vi "Read FRU.vi"(0 "Device In":T2, 1 "FRU Type":T5, 2 "FRU In":T4, 5 "i2c configuration in":T3, 7 "CSV Path":path, 9 "Unique FRU Data":T1, 11 "error in (no error)":errorcluster) -> (3 "FRU Out":T4, 4 "Device Out":T2, 6 "i2c configuration out":T3, 8 "Read Byte":u8[](array[numeric]) format="%02x", 14 "PASS":bool, 15 "error out":errorcluster)   [LabVIEW 2025]
uses:
  Type Definitions/FRU Information.ctl
  <vilib>/ni845x/ni845x.llb/ni845xControl.ctl
  <vilib>/ni845x/ni845x.llb/ni845xI2cConfiguration.ctl
  Type Definitions/FRU Type.ctl
  Type Definitions/Unique FRU Input.ctl
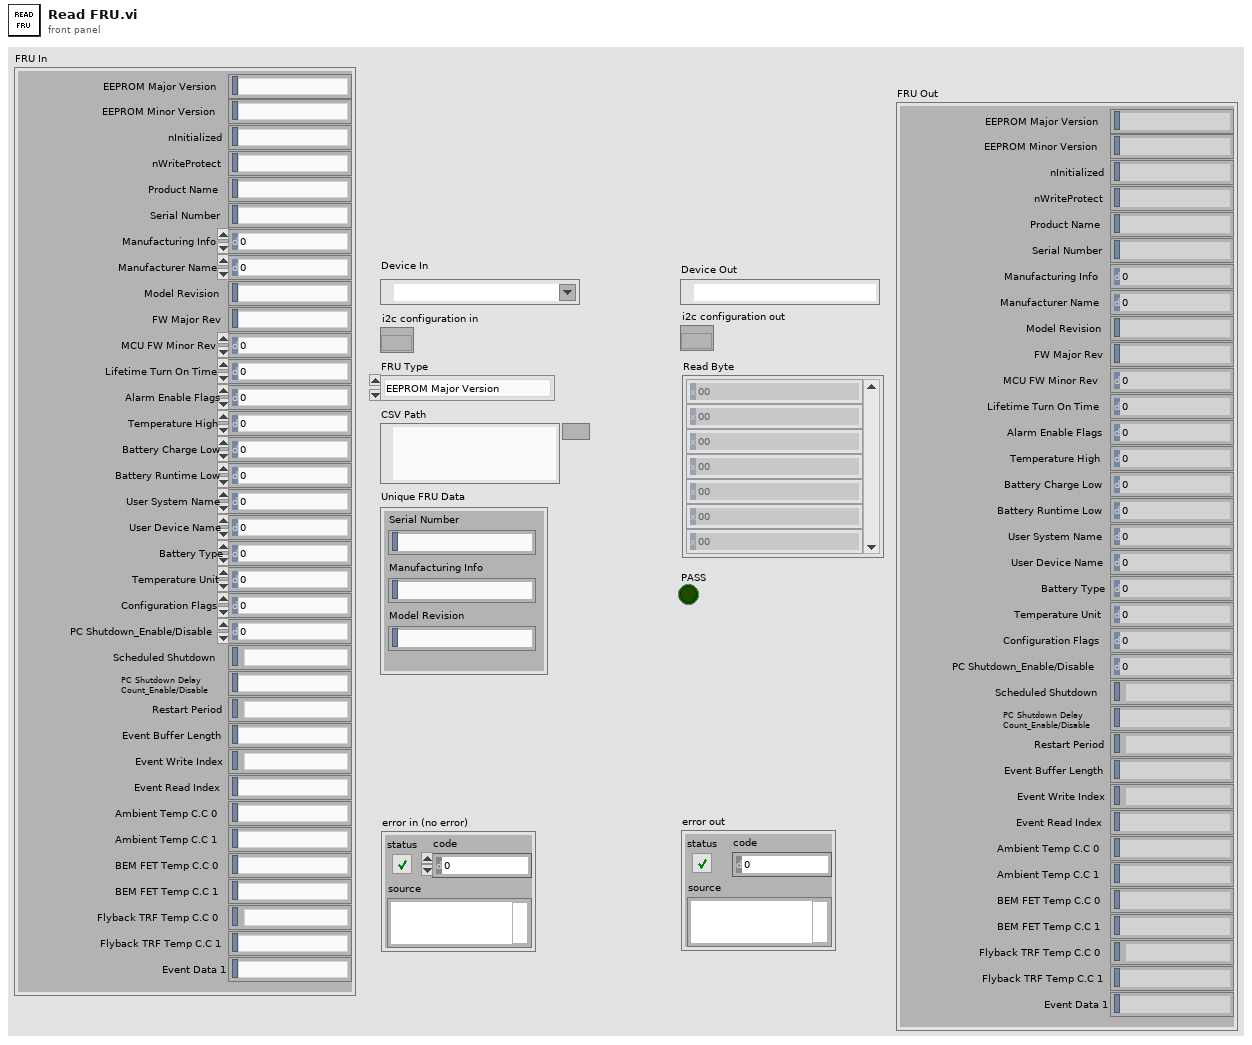
[diagram p1: front panel]
types:
  T1 = typedef "Unique FRU Input.ctl" = cluster{"Serial Number":string, "Manufacturing Info":string, "Model Revision":string}
  T2 = typedef "ni845xControl.ctl" = refnum<k21>
  T3 = typedef "ni845xI2cConfiguration.ctl" = refnum<k20>
  T4 = typedef "FRU Information.ctl" = cluster{"EEPROM Major Version":string, "EEPROM Minor Version":string, "nInitialized":string, "nWriteProtect":string, "Product Name":string, "Serial Number":string, "Manufacturing Info":u32, "Manufacturer Name":u32, "Model Revision":string, "FW Major Rev":string, "MCU FW Minor Rev":u32, "Lifetime Turn On Time":u32, "Alarm Enable Flags":u32, "Temperature High":u32, "Battery Charge Low":u32, "Battery Runtime Low":u32, "User System Name":u32, "User Device Name":u32, "Battery Type":u32, "Temperature Unit":u32, "Configuration Flags":u32, "PC Shutdown_Enable/Disable":u32, "Scheduled Shutdown":string, "PC Shutdown Delay Count_Enable/Disable":string, "Restart Period":string, "Event Buffer Length":string, "Event Write Index":string, "Event Read Index":string, "Ambient Temp C.C 0":string, "Ambient Temp C.C 1":string, "BEM FET Temp C.C 0":string, "BEM FET Temp C.C 1":string, "Flyback TRF Temp C.C 0":string, "Flyback TRF Temp C.C 1":string, "Event Data 1":string}
  T5 = typedef "FRU Type.ctl" = enum16{"EEPROM Major Version", "EEPROM Minor Version", "nInitialized", "nWriteProtect", "Product Name", "Serial Number", "Manufacturing Info", "Manufacturer Name", "Model Revision", "FW Major Rev", "MCU FW Minor Rev", "Lifetime Turn On Time", "Alarm Enable Flags", "Temperature High", "Battery Charge Low", "Battery Runtime Low", "User System Name", "User Device Name", "Battery Type", "Temperature Unit", "Configuration Flags", "PC Shutdown_Enable/Disable", "Scheduled Shutdown", "PC Shutdown Delay Count_Enable/Disable", "Restart Period", "Event Buffer Length", "Event Write Index", "Event Read Index", "Ambient Temp C.C 0", "Ambient Temp C.C 1", "BEM FET Temp C.C 0", "BEM FET Temp C.C 1", "Flyback TRF Temp C.C 0", "Flyback TRF Temp C.C 1", "Event Data", "EEPROM Unmodified"}
  T6 = typedef "I2C Data Cluster.ctl" = cluster{"Address Byte":u16, "Number of Bytes":u32, "Page Size in Bytes":u32, "Data Byte":u8[], "Write Delay Between Pages (ms)":u32}
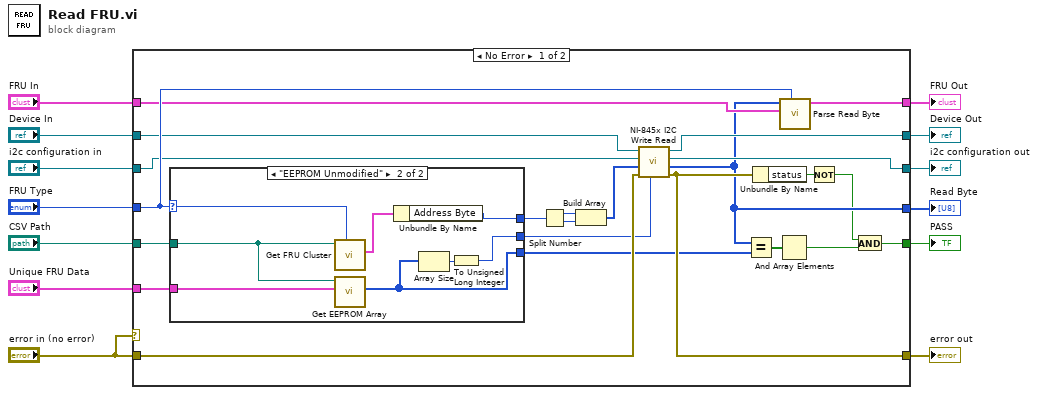
[diagram p0: block diagram]
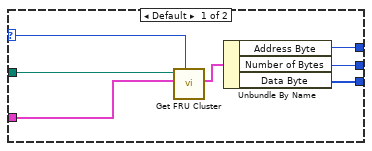
[diagram p2: hidden frame]
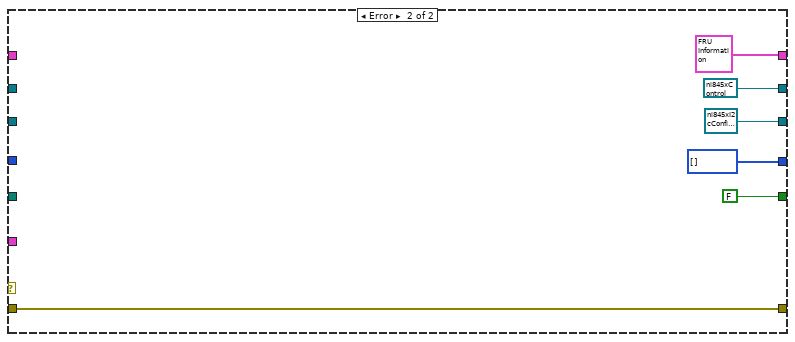
[diagram p3: hidden frame]
diagram:
  n1 = case shown="No Error" "error in (no error)" {
    tunnel: "FRU Type" -> [w36 _]
    tunnel: [w35 T3 refnum ("i2c configuration out")] -> w12
    tunnel: [w33 FALSE] -> w11
    tunnel: [w32 w57] -> w10
    tunnel: "FRU In" -> [w31 _]
    tunnel: [w30 T4 {"EEPROM Major Version"="", "EEPROM Minor Version"="", "nInitialized"="", "nWriteProtect"="", "Product Name"="", "Serial Number"="", "Manufacturing Info"=0, "Manufacturer Name"=0, "Model Revision"="", "FW Major Rev"="", "MCU FW Minor Rev"=0, "Lifetime Turn On Time"=0, "Alarm Enable Flags"=0, "Temperature High"=0, "Battery Charge Low"=0, "Battery Runtime Low"=0, "User System Name"=0, "User Device Name"=0, "Battery Type"=0, "Temperature Unit"=0, "Configuration Flags"=0, "PC Shutdown_Enable/Disable"=0, "Scheduled Shutdown"="", "PC Shutdown Delay Count_Enable/Disable"="", "Restart Period"="", "Event Buffer Length"="", "Event Write Index"="", "Event Read Index"="", "Ambient Temp C.C 0"="", "Ambient Temp C.C 1"="", "BEM FET Temp C.C 0"="", "BEM FET Temp C.C 1"="", "Flyback TRF Temp C.C 0"="", "Flyback TRF Temp C.C 1"="", "Event Data 1"=""} ("FRU Information Out")] -> w8
    tunnel: "error in (no error)" -> [w28 w57]
    tunnel: [w27 T2 refnum ("device reference out")] -> w7
    tunnel: "Device In" -> [w26 _]
    tunnel: "CSV Path" -> [w25 _]
    tunnel: "i2c configuration in" -> [w24 _]
    tunnel: [w23 u8[] [] ("read data")] -> w2
    tunnel: "Unique FRU Data" -> [w14 _]
    frame No Error {
      n2 = case shown="\"EEPROM Unmodified\"" w36 {
        selector: w36 -> [w42 w51]
        tunnel: w25 -> [w43 w48]
        tunnel: [w40 w49] -> w18
        tunnel: [w39 w46] -> w16
        tunnel: [w38 w45] -> w15
        tunnel: w14 -> [w37 w44]
        frame Default {
          n3 = call "Get FRU Cluster.vi"("FRU Type"=w42, "Unique FRU Input"=w37, "CSV Path"=w43) -> ("FRU Cluster"=w41:T6)  [unwired: 7 in, 1 out]
          n4 = Unbundle By Name(w41) -> ("Address Byte"=w40:u16, "Number of Bytes"=w39:u32, "Data Byte"=w38:u8[])
        }
        frame "EEPROM Unmodified" {
          n5 = call "Get FRU Cluster.vi"("FRU Type"=w51, "CSV Path"=w48) -> ("FRU Cluster"=w50:T6)  [unwired: 8 in, 1 out]
          n6 = call "Get EEPROM Array.vi"("Unique FRU Input"=w44, "CSV Path"=w48) -> ("EEPROM Array"=w45:u8[])  [unwired: 8 in, 1 out]
          n7 = Unbundle By Name(w50) -> ("Address Byte"=w49:u16)
          n8 = Array Size(array=w45) -> (size(s)=w47:i32)
          n9 = To Unsigned Long Integer(number=w47) -> (unsigned 32bit integer=w46:u32)
        }
      }
      n10 = Split Number(x=w18) -> (hi(x)=w20:u8, lo(x)=w19:u8)
      n11 = Build Array(w20, w19) -> (w17:u8[])
      n12 = call <vilib>:"NI-845x I2C Write Read.vi"("num bytes to read"=w16, "error in (no error)"=w28, "write data"=w17, "i2c configuration in"=w24, "device reference in"=w26) -> ("error out"=w32:errorcluster, "read data"=w23:u8[], "i2c configuration out"=w35:T3, "device reference out"=w27:T2)  [unwired: 3 in]
      n13 = Equal?(x=w23, y=w15) -> (x = y?=w29:bool[])
      n14 = Unbundle By Name(w32) -> ("status"=w22:bool)
      n15 = And Array Elements(Boolean array=w29) -> (logical AND=w34:bool)
      n16 = call "Parse Read Byte.vi"("Read Byte"=w23, "FRU Information In"=w31, "FRU Type"=w36) -> ("FRU Information Out"=w30:T4)  [unwired: 6 in, 1 out]
      n17 = Not(x=w22) -> (.not. x?=w21:bool)
      n18 = And(x=w21, y=w34) -> (x .and. y?=w33:bool)
    }
    frame Error {
    }
  }
  "i2c configuration out" <- w12
  "PASS" <- w11
  "error out" <- w10
  "FRU Out" <- w8
  "Device Out" <- w7
  "Read Byte" <- w2
